vi "date save to excel.vi"() -> (3 "concatenated string":string)   [LabVIEW 2014]
panel:
  out "Path Format":path
  out "Minute":string
  out "Hour":string
  out "Day":string
  out "Month":string
  out "Year":string
  in  "Path to SAVE":path
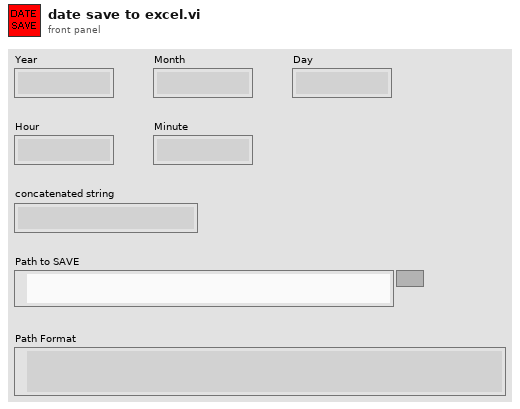
[diagram p1: front panel]
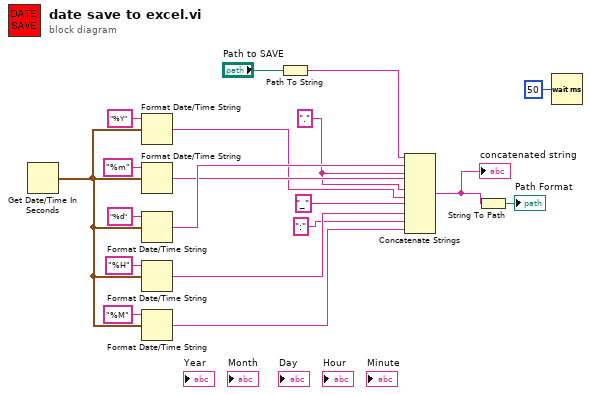
[diagram p0: block diagram]
diagram:
  w2 = "." ("string")
  n1 = Get Date/Time In Seconds() -> (seconds since 1Jan1904=w19:timestamp)
  n2 = Format Date/Time String(time format string (%c)="%Y", seconds (now)=w19) -> (date/time string=w1:string)  [unwired: 1 in]
  n3 = Format Date/Time String(time format string (%c)="%m", seconds (now)=w19) -> (date/time string=w3:string)  [unwired: 1 in]
  n4 = Format Date/Time String(time format string (%c)="%d", seconds (now)=w19) -> (date/time string=w4:string)  [unwired: 1 in]
  n5 = Format Date/Time String(time format string (%c)="%H", seconds (now)=w19) -> (date/time string=w9:string)  [unwired: 1 in]
  n6 = Format Date/Time String(time format string (%c)="%M", seconds (now)=w19) -> (date/time string=w7:string)  [unwired: 1 in]
  n7 = Path To String(path="Path to SAVE") -> (string=w5:string)
  n8 = Concatenate Strings(w5, w4, w2, w3, w2, w1, "_" ("string"), w9, ":" ("string"), w7) -> (w11:string)
  "concatenated string" <- w11
  n9 = String To Path(string=w11) -> (path=→"Path Format":path)
  n10 = Wait (ms)(milliseconds to wait=u32 50) -> ()  [unwired: 1 out]
